vi "Drive distance with encoders.vi"(8 "error in (no error)":errorcluster, 11 "Wanted Distance":dbl) -> (0 "error out":errorcluster)   [LabVIEW 2017]
uses:
  Public/Documents/Cross The Road Electronics/Phoenix-LabVIEW/Motor Controller/Get/CTRE_Phoenix_MotorController_GetSelectedSensorData.vi
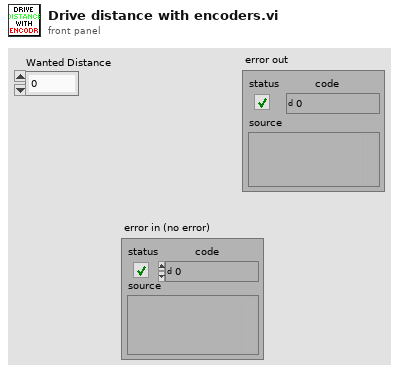
[diagram p1: front panel]
types:
  T1 = typedef "WPI_MotorControlDeviceRef.ctl" = cluster{"DeviceStatus":errorcluster, "Type":T2, "PWM":cluster{"PWM Channel":T3, "DeadBand":T4}, "CAN":cluster{"Device Number":u8, "SetOutput VI Ref":variant, "GetOutput VI Ref":variant, "Enable VI Ref":variant, "Disable VI Ref":variant, "Data":variant}, "Invert":bool, "DIO PWM":cluster{"PWM \"Enable\" Channel":T3, "DIOChannel":T5, "PWM Rate":dbl}}
  T2 = typedef "WPI_MotorControlType.ctl" = enum16{"PWM", "CAN", "DIO PWM"}
  T3 = typedef "FPGA_DIOPWMChannel.ctl" = enum8{"PWM 0", "PWM 1", "PWM 2", "PWM 3", "PWM 4", "PWM 5", "PWM 6", "PWM 7", "PWM 8", "PWM 9", "PWM MXP 0", "PWM MXP 1", "PWM MXP 2", "PWM MXP 3", "PWM MXP 4", "PWM MXP 5", "PWM MXP 6", "PWM MXP 7", "PWM MXP 8", "PWM MXP 9", "Invalid"}
  T4 = typedef "WPI_PWMDeadband.ctl" = cluster{"Name":string, "maxPositivePwm":i32, "minPositivePwm":i32, "centerPwm":i32, "maxNegativePwm":i32, "minNegativePwm":i32, "angularRange":u16}
  T5 = typedef "FPGA_DIOChannel.ctl" = enum8{"DIO 0", "DIO 1", "DIO 2", "DIO 3", "DIO 4", "DIO 5", "DIO 6", "DIO 7", "DIO 8", "DIO 9", "DIO MXP 0", "DIO MXP 1", "DIO MXP 2", "DIO MXP 3", "DIO MXP 4", "DIO MXP 5", "DIO MXP 6", "DIO MXP 7", "DIO MXP 8", "DIO MXP 9", "DIO MXP 10", "DIO MXP 11", "DIO MXP 12", "DIO MXP 13", "DIO MXP 14", "DIO MXP 15", "SPI Port CS1", "SPI Port CS2", "SPI Port CS3", "SPI Port MISO", "SPI Port MOSI", "Invalid"}
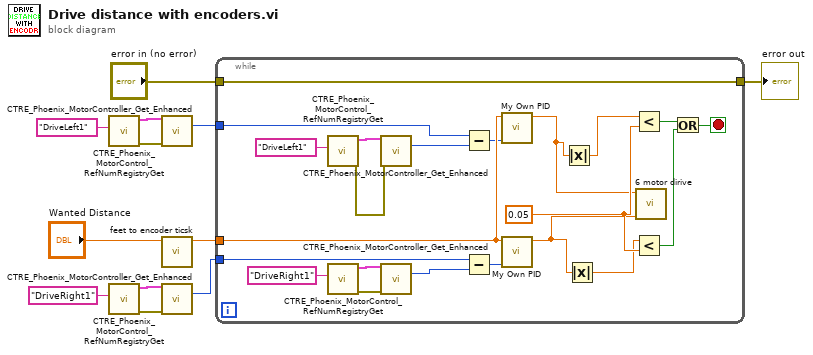
[diagram p0: block diagram]
diagram:
  n1 = call "CTRE_Phoenix_MotorControl_RefNumRegistryGet.vi"("refnum name"="DriveLeft1") -> ("error out"=w6:errorcluster, "PhoenixMotorControlDevRef"=w10:T1)  [unwired: 9 in]
  n2 = call "CTRE_Phoenix_MotorControl_RefNumRegistryGet.vi"("refnum name"="DriveRight1") -> ("error out"=w5:errorcluster, "PhoenixMotorControlDevRef"=w7:T1)  [unwired: 9 in]
  n3 = call-poly "CTRE_Phoenix_MotorController_Get_Enhanced.vi"("PhoenixMotorControlDevRef"=w10, "error in"=w6) -> ("Position (Raw Sensor Units)"=w4:i32)  [unwired: 10 in, 3 out]
  n4 = call "feet to encoder ticsk.vi"("Distance in feet wanted"="Wanted Distance") -> ("Encoder Ticks"=w11:dbl)  [unwired: 10 in]
  n5 = call-poly "CTRE_Phoenix_MotorController_Get_Enhanced.vi"("PhoenixMotorControlDevRef"=w7, "error in"=w5) -> ("Position (Raw Sensor Units)"=w3:i32)  [unwired: 10 in, 3 out]
  n6 = while {
    tunnel: w11 -> [w34]
    tunnel: w4 -> [w27]
    tunnel: w3 -> [w25]
    tunnel: [w17] -> w2
    tunnel: "error in (no error)" -> [w17]
    stop <- w21 stop-if-true
    w20 = 0.05
    n7 = call "CTRE_Phoenix_MotorControl_RefNumRegistryGet.vi"("refnum name"="DriveLeft1") -> ("error out"=w32:errorcluster, "PhoenixMotorControlDevRef"=w28:T1)  [unwired: 9 in]
    n8 = call "CTRE_Phoenix_MotorControl_RefNumRegistryGet.vi"("refnum name"="DriveRight1") -> ("error out"=w33:errorcluster, "PhoenixMotorControlDevRef"=w31:T1)  [unwired: 9 in]
    n9 = call-poly "CTRE_Phoenix_MotorController_Get_Enhanced.vi"("PhoenixMotorControlDevRef"=w28, "error in"=w32) -> ("Position (Raw Sensor Units)"=w26:i32)  [unwired: 10 in, 3 out]
    n10 = call-poly "CTRE_Phoenix_MotorController_Get_Enhanced.vi"("PhoenixMotorControlDevRef"=w31, "error in"=w33) -> ("Position (Raw Sensor Units)"=w24:i32)  [unwired: 10 in, 3 out]
    n11 = Subtract(x=w27, y=w26) -> (x-y=w23:i32)
    n12 = Subtract(x=w25, y=w24) -> (x-y=w22:i32)
    n13 = call "My Own PID.vi"("Current Input"=w23, "Wanted End"=w34) -> ("Output"=w14:dbl)  [unwired: 9 in]
    n14 = call "My Own PID.vi"("Current Input"=w22, "Wanted End"=w34) -> ("Output"=w16:dbl)  [unwired: 9 in]
    n15 = Absolute Value(x=w14) -> (abs(x)=w13:dbl)
    n16 = Absolute Value(x=w16) -> (abs(x)=w15:dbl)
    n17 = Less?(x=w13, y=w20) -> (x < y?=w19:bool)
    n18 = Less?(x=w15, y=w20) -> (x < y?=w18:bool)
    n19 = call "6 motor dirive.vi"("Right Joystick"=w16, "Left Joystick"=w14) -> ()  [unwired: 10 in]
    n20 = Or(x=w19, y=w18) -> (x .or. y?=w21:bool)
  }
  "error out" <- w2
